vi "query.vi"(8 "error in (no error)":errorcluster, 10 "write buffer":string, 11 "VISA resource name":refnum<visa-resource-name>) -> (0 "error out":errorcluster, 2 "substring":string, 3 "VISA resource name out":refnum<visa-resource-name>)   [LabVIEW 2013]
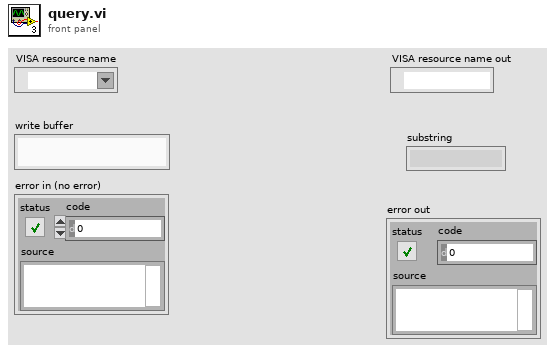
[diagram p1: front panel]
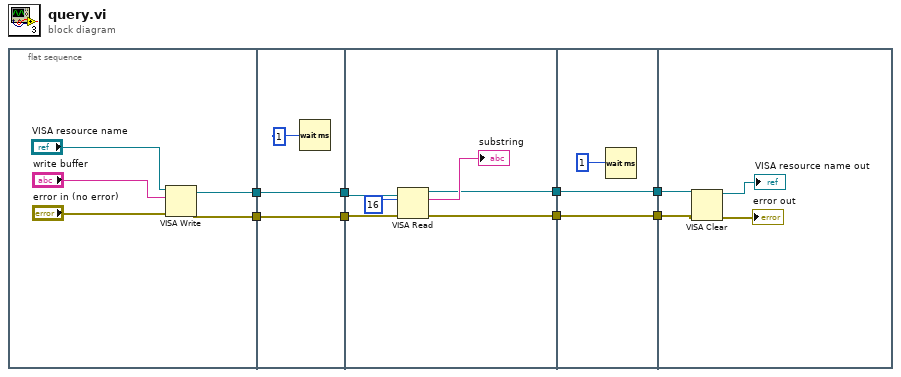
[diagram p0: block diagram]
diagram:
  n1 = flat-sequence {
    tunnel: [w13] -> w8
    tunnel: [w12] -> w7
    tunnel: w8 -> [w16]
    tunnel: w7 -> [w15]
    tunnel: [w16] -> w6
    tunnel: [w15] -> w5
    tunnel: w6 -> [w21]
    tunnel: w5 -> [w20]
    tunnel: [w18] -> w4
    tunnel: [w17] -> w2
    tunnel: w4 -> [w25]
    tunnel: [w25] -> w3
    tunnel: w2 -> [w24]
    tunnel: [w24] -> w1
    tunnel: w3 -> [w29]
    tunnel: w1 -> [w28]
    frame #0 {
      n2 = VISA Write(VISA resource name="VISA resource name", write buffer="write buffer", error in (no error)="error in (no error)") -> (VISA resource name out=w13:refnum<visa-resource-name>, error out=w12:errorcluster)  [unwired: 1 out]
    }
    frame #1 {
      n3 = Wait (ms)(milliseconds to wait=u32 1) -> ()  [unwired: 1 out]
    }
    frame #2 {
      n4 = VISA Read(VISA resource name=w21, byte count=u32 16, error in (no error)=w20) -> (VISA resource name out=w18:refnum<visa-resource-name>, read buffer=→"substring":string, error out=w17:errorcluster)  [unwired: 1 out]
    }
    frame #3 {
      n5 = Wait (ms)(milliseconds to wait=u32 1) -> ()  [unwired: 1 out]
    }
    frame #4 {
      n6 = VISA Clear(VISA resource name=w29, error in (no error)=w28) -> (VISA resource name out=→"VISA resource name out":refnum<visa-resource-name>, error out=→"error out":errorcluster)
    }
  }
